vi "get_S12CON.vi"(8 "error in (no error)":errorcluster caption="错误输入（无错误）", 11 "StepMotor输入":refnum<class "StepMotor.lvclass">) -> (0 "error out":errorcluster caption="错误输出", 2 "S12CON寄存器设置":T1={"S2传感器上升沿绑定动作"=0, "S2传感器下降沿绑定动作"=1, "S1传感器上升沿绑定动作"=2, "S1传感器下降沿绑定动作"=3} {"S1传感器下降沿绑定动作" items=["无动作，无状态通知"=0, "无动作，有通知"=1, "负向连续运行"=2, "减速直到停止"=3, "紧急停止"=4, "负向相对位移控制"=5, "绝对位置清零"=6, "绝对位置清零+相对位移控制"=7, "换向相对位移控制"=9, "正向连续运行"=10, "绝对位置清零+减速直到停止"=11, "绝对位置清零+紧急停止"=12, "正向相对位移控制"=13, "换向连续运行"=14, "脱机"=15]; "S1传感器上升沿绑定动作" items=["无动作，无状态通知"=0, "无动作，有通知"=1, "负向连续运行"=2, "减速直到停止"=3, "紧急停止"=4, "负向相对位移控制"=5, "绝对位置清零"=6, "绝对位置清零+相对位移控制"=7, "换向相对位移控制"=9, "正向连续运行"=10, "绝对位置清零+减速直到停止"=11, "绝对位置清零+紧急停止"=12, "正向相对位移控制"=13, "换向连续运行"=14, "脱机"=15]; "S2传感器下降沿绑定动作" items=["无动作，无状态通知"=0, "无动作，有通知"=1, "负向连续运行"=2, "减速直到停止"=3, "紧急停止"=4, "负向相对位移控制"=5, "绝对位置清零"=6, "绝对位置清零+相对位移控制"=7, "换向相对位移控制"=9, "正向连续运行"=10, "绝对位置清零+减速直到停止"=11, "绝对位置清零+紧急停止"=12, "正向相对位移控制"=13, "换向连续运行"=14, "脱机"=15]; "S2传感器上升沿绑定动作" items=["无动作，无状态通知"=0, "无动作，有通知"=1, "负向连续运行"=2, "减速直到停止"=3, "紧急停止"=4, "负向相对位移控制"=5, "绝对位置清零"=6, "绝对位置清零+相对位移控制"=7, "换向相对位移控制"=9, "正向连续运行"=10, "绝对位置清零+减速直到停止"=11, "绝对位置清零+紧急停止"=12, "正向相对位移控制"=13, "换向连续运行"=14, "脱机"=15]}, 3 "StepMotor输出":refnum<class "StepMotor.lvclass">)   [LabVIEW 2016, in "MotionControl_UFO_3DOF.lvlib" / "StepMotor.lvclass"]
uses:
  <userlib>/MotionControl_UFO_3DOF/StepMotor/StepMotor.lvclass
  <userlib>/MotionControl_UFO_3DOF/StepMotor/StepMotor.lvclass/StepMotor.ctl
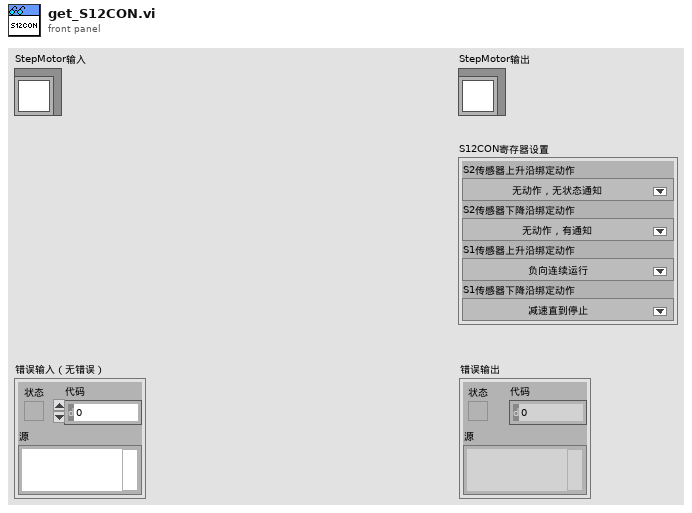
[diagram p1: front panel]
types:
  T1 = cluster{"S2传感器上升沿绑定动作":u32, "S2传感器下降沿绑定动作":u32, "S1传感器上升沿绑定动作":u32, "S1传感器下降沿绑定动作":u32}
  T2 = typedef "MotionControl_UFO_3DOF.lvlib/StepMotor.lvclass/S12CON.ctl" = cluster{"S2传感器上升沿绑定动作":u32, "S2传感器下降沿绑定动作":u32, "S1传感器上升沿绑定动作":u32, "S1传感器下降沿绑定动作":u32}
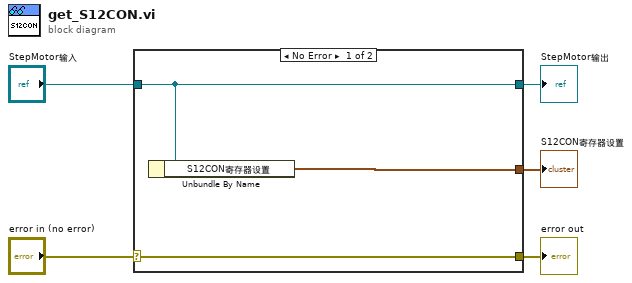
[diagram p0: block diagram]
diagram:
  n1 = case shown="No Error" "error in (no error)" {
    selector: "error in (no error)" -> [w8 w9]
    tunnel: [w8 w9] -> w4
    tunnel: [w7 w10] -> w2
    tunnel: "StepMotor输入" -> [w7 w10]
    tunnel: [w6 _] -> w1
    frame No Error {
      n2 = Unbundle By Name(w7) -> ("S12CON寄存器设置"=w6:T2)
    }
    frame Error {
    }
  }
  "error out" <- w4
  "StepMotor输出" <- w2
  "S12CON寄存器设置" <- w1
